vi "Labstep tester.vi"() -> ()   [LabVIEW 2015]
panel:
  in  "API Key":string="ZDNlNzY2YTYwNjk2YjY0Y2E4OGZhMGNiMDYxMWJkZjVjNWMwMjMzOQ=="
  in  "Name of LAG SIM user":string
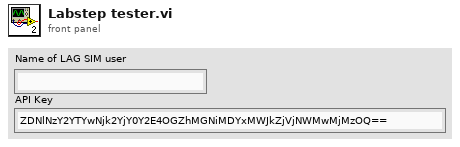
[diagram p1: front panel]
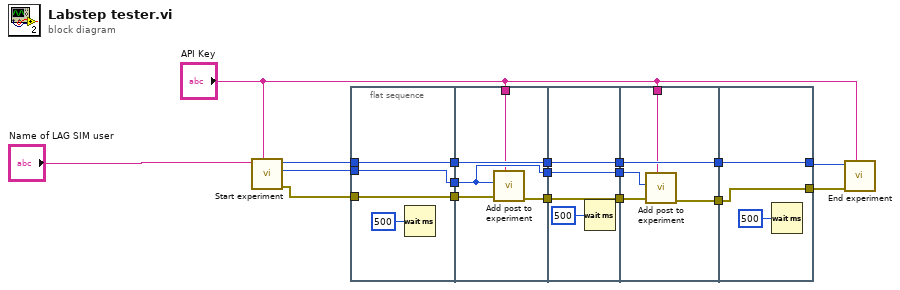
[diagram p0: block diagram]
diagram:
  n1 = call "Start experiment.vi"("API Key"="API Key", "Name of LAG SIM user"="Name of LAG SIM user") -> ("error out"=w5:errorcluster, "Thread ID"=w11:i32, "Experiment ID"=w17:i32)  [unwired: 7 in]
  n2 = flat-sequence {
    tunnel: w17 -> [w22]
    tunnel: [w22] -> w15
    tunnel: w11 -> [w20]
    tunnel: [w20] -> w10
    tunnel: [w19] -> w6
    tunnel: w5 -> [w19]
    tunnel: w15 -> [w27]
    tunnel: [w27] -> w14
    tunnel: w10 -> [w26]
    tunnel: [w26] -> w8
    tunnel: "API Key" -> [w25]
    tunnel: w6 -> [w24]
    tunnel: [w23] -> w3
    tunnel: w14 -> [w31]
    tunnel: [w31] -> w13
    tunnel: [w29] -> w9
    tunnel: w8 -> [w29]
    tunnel: [w28] -> w4
    tunnel: w3 -> [w28]
    tunnel: w13 -> [w36]
    tunnel: [w36] -> w12
    tunnel: w9 -> [w35]
    tunnel: "API Key" -> [w34]
    tunnel: w4 -> [w33]
    tunnel: [w32] -> w2
    tunnel: [w39] -> w16
    tunnel: w12 -> [w39]
    tunnel: w2 -> [w37]
    tunnel: [w37] -> w1
    frame #0 {
      n3 = Wait (ms)(milliseconds to wait=u32 500) -> ()  [unwired: 1 out]
    }
    frame #1 {
      n4 = call "Add post to experiment.vi"("API Key"=w25, "error in"=w24, "Thraed ID"=w26) -> ("error out"=w23:errorcluster)  [unwired: 8 in]
    }
    frame #2 {
      n5 = Wait (ms)(milliseconds to wait=u32 500) -> ()  [unwired: 1 out]
    }
    frame #3 {
      n6 = call "Add post to experiment.vi"("API Key"=w34, "error in"=w33, "Thraed ID"=w35) -> ("error out"=w32:errorcluster)  [unwired: 8 in]
    }
    frame #4 {
      n7 = Wait (ms)(milliseconds to wait=u32 500) -> ()  [unwired: 1 out]
    }
  }
  n8 = call "End experiment.vi"("API Key"="API Key", "error in"=w1, "Experiment ID"=w16) -> ()  [unwired: 8 in, 1 out]
